vi "check_counter_date.vi"(8 "error in":errorcluster) -> (0 "error out":errorcluster)   [LabVIEW 2012]
uses:
  <vilib>/addons/database/Connection.llb/Conn Execute.vi
  <vilib>/addons/database/Recordset.llb/Rec Fetch Recordset Data (R).vi
  <vilib>/addons/database/Recordset.llb/Rec Destroy - Connection.vi
  <vilib>/addons/database/_DB Variant To Data/Database Variant To Data.xnode
  <vilib>/addons/database/NI_Database_API.lvlib
panel:
  out "Test Server":bool
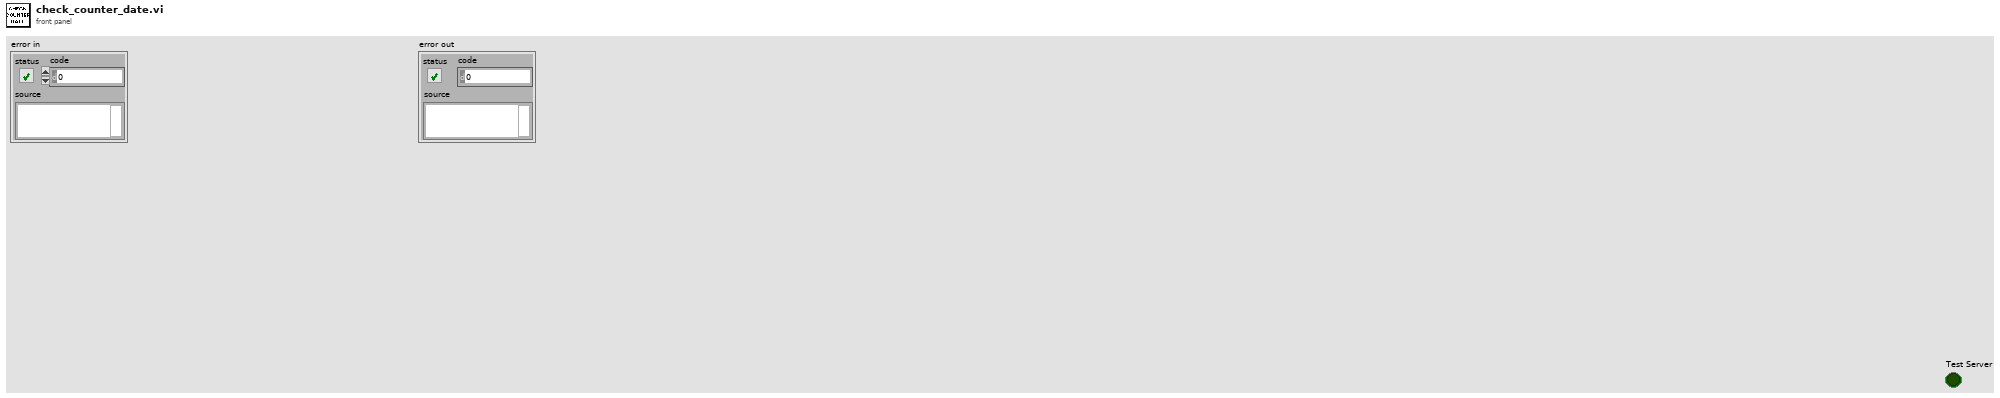
[diagram p1: front panel]
types:
  T1 = typedef "NI_Database_API.lvlib/Conn ObjectReference.ctl" = refnum<k1>
  T2 = typedef "NI_Database_API.lvlib/Rec ObjectReference.ctl" = refnum<k1>
  T3 = cluster{"Integer Time":i64, "Integer Timestamp":i64, "Integer Timestamp":i64, "Integer Timestamp":i64, "Integer Timestamp":i64}
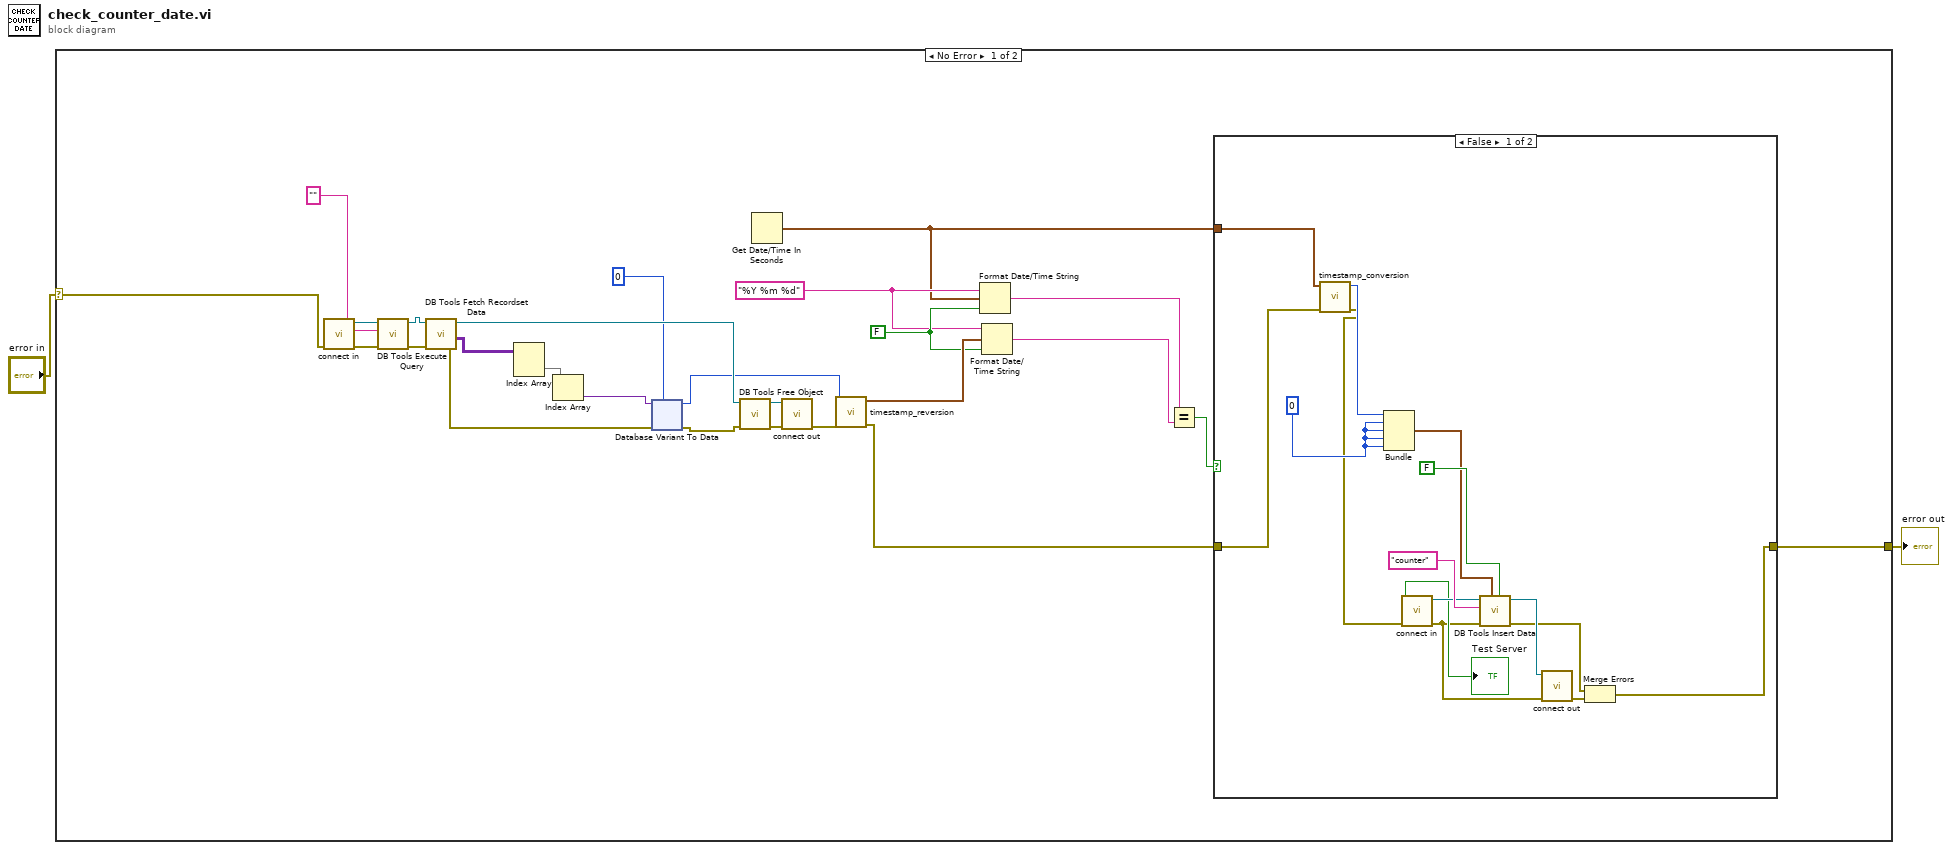
[diagram p0: block diagram]
diagram:
  n1 = case shown="No Error" "error in" {
    selector: "error in" -> [w16 w77]
    tunnel: [w4 w77] -> w1
    frame No Error {
      w6 = "%Y %m %d" ("time format string (%c)")
      w9 = FALSE ("UTC format")
      n2 = call "connect in.vi"("error in (no error)"=w16) -> ("error out"=w27:errorcluster, "Database Connection"=w23:T1)  [unwired: 6 in, 1 out]
      n3 = call-poly <vilib>:"DB Tools Execute Query.vi"("error in (no error)"=w27, "SQL query"="", "connection reference"=w23) -> ("error out"=w28:errorcluster, "recordset reference"=w24:T2)  [unwired: 5 in]
      n4 = call-poly <vilib>:"DB Tools Fetch Recordset Data.vi"("error in (no error)"=w28, "recordset reference"=w24) -> ("error out"=w20:errorcluster, "recordset data"=w26:variant[][], "recordset reference out"=w18:T2)  [unwired: 3 in]
      n5 = Index Array(array=w26) -> (element=w25:variant[])  [unwired: 2 in]
      n6 = Index Array(array=w25) -> (element=w22:variant)  [unwired: 1 in]
      n7 = xnode "Database Variant To Data"("database variant"=w22, "error in (no error)"=w20, "type"=i64 0 ("Integer Timestamp")) -> ("data"=w13:i64, "error out"=w19:errorcluster)
      n8 = call-poly <vilib>:"DB Tools Free Object.vi"("error in (no error)"=w19, "recordset reference"=w18) -> ("error out"=w21:errorcluster, "connection reference"=w17:T1)  [unwired: 8 in]
      n9 = Get Date/Time In Seconds() -> (seconds since 1Jan1904=w3:timestamp)
      n10 = call "connect out.vi"("error in (no error)"=w21, "connection reference"=w17) -> ("error out"=w12:errorcluster)  [unwired: 9 in]
      n11 = call "timestamp_reversion.vi"("error in (no error)"=w12, "Integer Timestamp"=w13) -> ("error out"=w5:errorcluster, "time stamp"=w10:timestamp)  [unwired: 7 in]
      n12 = Format Date/Time String(time format string (%c)=w6, seconds (now)=w3, UTC format=w9) -> (date/time string=w7:string)
      n13 = Format Date/Time String(time format string (%c)=w6, seconds (now)=w10, UTC format=w9) -> (date/time string=w8:string)
      n14 = Equal?(x=w7, y=w8) -> (x = y?=w11:bool)
      n15 = case shown="False" w11 {
        tunnel: w5 -> [w40 w44]
        tunnel: [w29 w44] -> w4
        tunnel: w3 -> [w42 _]
        frame False {
          w43 = i64 0 ("Integer Timestamp")
          n16 = call "timestamp_conversion.vi"("error in (no error)"=w40, "Time Stamp"=w42) -> ("error out"=w30:errorcluster, "Integer Time"=w41:i64)  [unwired: 7 in]
          n17 = Bundle("Integer Time"=w41, "Integer Timestamp"=w43, "Integer Timestamp"=w43, "Integer Timestamp"=w43, "Integer Timestamp"=w43) -> (w31:T3)  [unwired: 1 in]
          n18 = call "connect in.vi"("error in (no error)"=w30) -> ("error out"=w33:errorcluster, "Database Connection"=w38:T1, "Test Server"=→"Test Server":bool)  [unwired: 6 in]
          n19 = call <vilib>:"DB Tools Insert Data.vi"("create table? (F)"=FALSE, "data"=w31, "error in (no error)"=w33, "table"="counter", "connection reference"=w38) -> ("error out"=w34:errorcluster, "connection reference out"=w37:T1)  [unwired: 5 in]
          n20 = call "connect out.vi"("error in (no error)"=w33, "connection reference"=w37) -> ("error out"=w32:errorcluster)  [unwired: 9 in]
          n21 = Merge Errors(w34, w32) -> (w29:errorcluster)
        }
        frame True {
        }
      }
    }
    frame Error {
    }
  }
  "error out" <- w1
